vi "WC_Drive_Read Profile Array from File.vi"(7 "Profile Path":path=path "/home/lvuser/mp.csv", 8 "Error":errorcluster, 9 "Select":T1, 11 "Point Array":T2) -> (0 "Error Out":errorcluster, 3 "Point Array Out":T2)   [LabVIEW 2016]
uses:
  RoboRio code/TypeDef/CLUSTER_Drive_Motion Profile Arrays.ctl
  RoboRio code/TypeDef/CLUSTER_Drive_Point Specification.ctl
  Dashboard/TypeDefs/ENUM_Profile File Function Select.ctl
  <vilib>/Utility/file.llb/Read Delimited Spreadsheet (DBL).vi
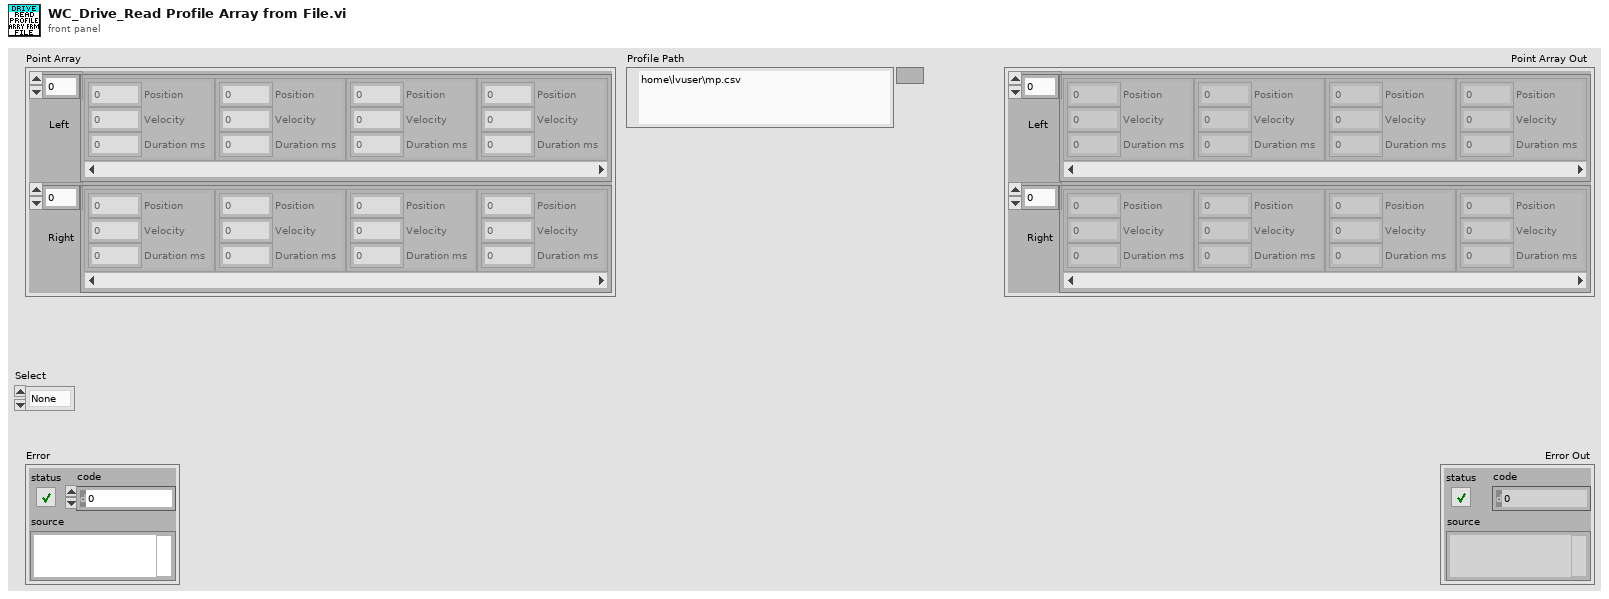
[diagram p1: front panel]
types:
  T1 = typedef "ENUM_Profile File Function Select.ctl" = enum16{"None", "Left", "Right", "Both"}
  T2 = typedef "CLUSTER_Drive_Motion Profile Arrays.ctl" = cluster{"Left":T3[], "Right":T3[]}
  T3 = typedef "CLUSTER_Drive_Point Specification.ctl" = cluster{"Position":dbl, "Velocity":dbl, "Duration ms":u8}
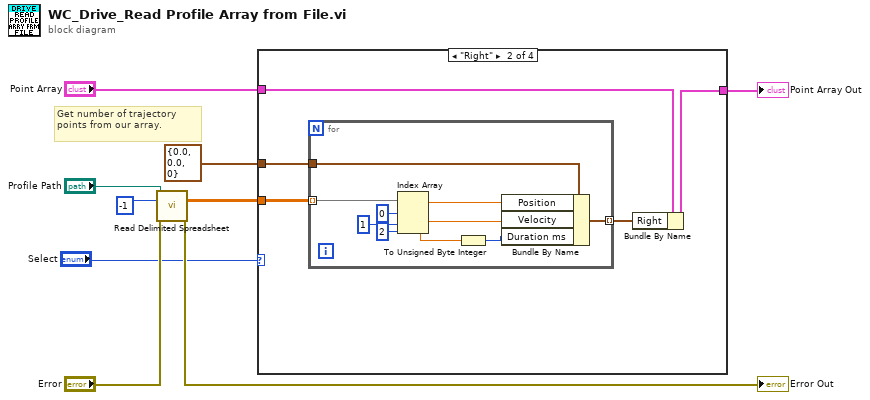
[diagram p0: block diagram]
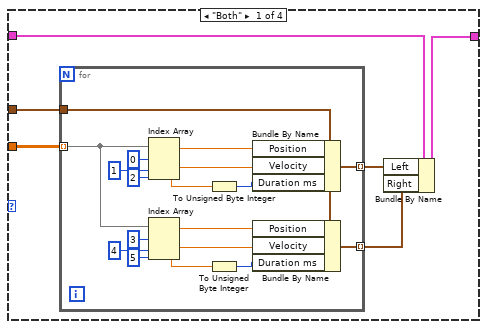
[diagram p2: hidden frame]
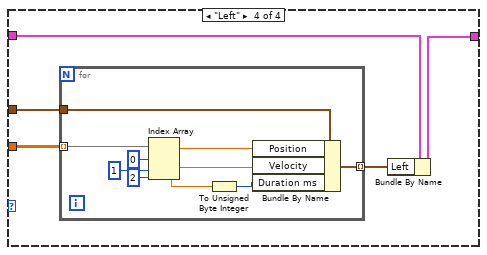
[diagram p4: hidden frame]
diagram:
  # "Get number of trajectory points from our array."
  n1 = call-poly <vilib>:"Read Delimited Spreadsheet.vi"("file path (dialog if empty)"="Profile Path", "number of rows (all:-1)"=-1, "error in (no error)"="Error") -> ("all rows"=w7:dbl[][], "error out"=→"Error Out":errorcluster)  [unwired: 7 in, 4 out]
  n2 = case shown="\"Right\"" "Select" {
    tunnel: w7 -> [w15 w38 _ w54]
    tunnel: T3 {"Position"=0.0, "Velocity"=0.0, "Duration ms"=0} -> [w14 w37 _ w53]
    tunnel: [w11 w35 w49 w51] -> w3
    tunnel: "Point Array" -> [w10 w34 w49 w50]
    frame "Both" {
      n3 = for {
        tunnel: w15 -> [w17] mode=indexing
        tunnel: w14 -> [w18]
        tunnel: [w26] -> w12 mode=indexing
        tunnel: [w16] -> w13 mode=indexing
        n4 = Index Array(array=w17, index #1=0 ("index"), index #2=1 ("index"), index #3=2 ("index")) -> (element #1=w29:dbl, element #2=w30:dbl, element #3=w28:dbl)
        n5 = Index Array(array=w17, index #1=3 ("index"), index #2=4 ("index"), index #3=5 ("index")) -> (element #1=w23:dbl, element #2=w22:dbl, element #3=w24:dbl)
        n6 = To Unsigned Byte Integer(number=w28) -> (unsigned 8bit integer=w27:u8)
        n7 = To Unsigned Byte Integer(number=w24) -> (unsigned 8bit integer=w25:u8)
        n8 = Bundle By Name(cluster=w18, "Position"=w29, "Velocity"=w30, "Duration ms"=w27) -> (w26:T3)
        n9 = Bundle By Name(cluster=w18, "Position"=w23, "Velocity"=w22, "Duration ms"=w25) -> (w16:T3)
      }
      n10 = Bundle By Name(cluster=w10, "Left"=w12, "Right"=w13) -> (w11:T2)
    }
    frame "Right" {
      n11 = for {
        tunnel: w38 -> [w39] mode=indexing
        tunnel: w37 -> [w40]
        tunnel: [w41] -> w36 mode=indexing
        n12 = Index Array(array=w39, index #1=0 ("index"), index #2=1 ("index"), index #3=2 ("index")) -> (element #1=w44:dbl, element #2=w45:dbl, element #3=w43:dbl)
        n13 = To Unsigned Byte Integer(number=w43) -> (unsigned 8bit integer=w42:u8)
        n14 = Bundle By Name(cluster=w40, "Position"=w44, "Velocity"=w45, "Duration ms"=w42) -> (w41:T3)
      }
      n15 = Bundle By Name(cluster=w34, "Right"=w36) -> (w35:T2)
    }
    frame "None" {
    }
    frame "Left" {
      n16 = for {
        tunnel: w54 -> [w55] mode=indexing
        tunnel: w53 -> [w56]
        tunnel: [w57] -> w52 mode=indexing
        n17 = Index Array(array=w55, index #1=0 ("index"), index #2=1 ("index"), index #3=2 ("index")) -> (element #1=w60:dbl, element #2=w61:dbl, element #3=w59:dbl)
        n18 = To Unsigned Byte Integer(number=w59) -> (unsigned 8bit integer=w58:u8)
        n19 = Bundle By Name(cluster=w56, "Position"=w60, "Velocity"=w61, "Duration ms"=w58) -> (w57:T3)
      }
      n20 = Bundle By Name(cluster=w50, "Left"=w52) -> (w51:T2)
    }
  }
  "Point Array Out" <- w3
